vi "Update Slot Configuration.vi"(8 "error in (no error)":errorcluster, 9 "Card Position":T1[](array[typedef]) {"Slot #" max=15}, 10 "Card Name":string[](array[string]), 11 "Slot Configuration in":refnum<vi>) -> (0 "error out":errorcluster, 3 "Slot Configuration out":refnum<vi>)   [LabVIEW 2014, in "SLSC configuration System Explorer.lvlib"]
uses:
  SLSC configuration System Explorer.lvlib
  Type Defs/Card Position.ctl
  Example/SPI Utility/Slot #.ctl
  <vilib>/Utility/miscctls.llb/LVRowAndColumnTypeDef.ctl
  Shared/Constants.vi
  Shared/SLSC configuration Shared.lvlib
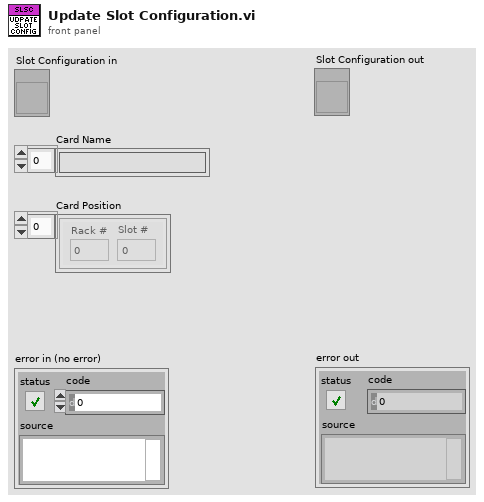
[diagram p1: front panel]
types:
  T1 = typedef "SLSC configuration Shared.lvlib/Card Position.ctl" = cluster{"Rack #":u8, "Slot #":T2}
  T2 = typedef "SLSC configuration Shared.lvlib/Slot #.ctl" = u8
  T3 = typedef "LVRowAndColumnTypeDef.ctl" = cluster{"Row":i32, "Column":i32}
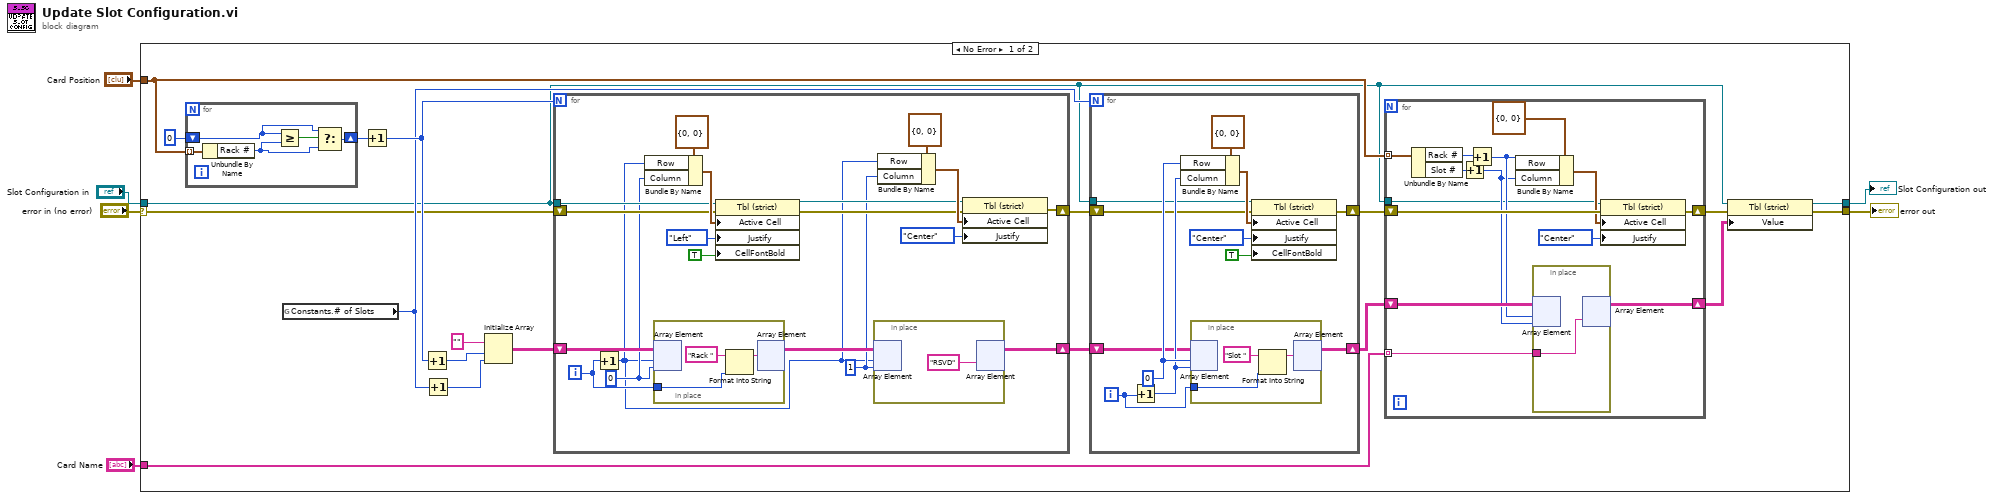
[diagram p0: block diagram]
diagram:
  n1 = case shown="No Error" "error in (no error)" {
    selector: "error in (no error)" -> [w12 w85]
    tunnel: "Card Position" -> [w23 _]
    tunnel: "Card Name" -> [w22 _]
    tunnel: [w10 w85] -> w1
    tunnel: "Slot Configuration in" -> [w7 w86]
    tunnel: [w8 w86] -> w2
    frame No Error {
      n2 = for {
        tunnel: w23 -> [w80] mode=indexing
        shift-right: [w81] -> w20
        shift-left: u8 0 ("Rack #") -> [w83]
        n3 = Unbundle By Name(w80) -> ("Rack #"=w82:u8)
        n4 = Greater Or Equal?(x=w83, y=w82) -> (x >= y?=w84:bool)
        n5 = Select(t=w83, s=w84, f=w82) -> (s? t:f=w81:u8)
      }
      n6 = global read "Constants.vi" "Constants.# of Slots"() -> (w13:u8)
      n7 = Increment(x=w20) -> (x+1=w19:u8)
      n8 = Increment(x=w19) -> (x+1=w24:u8)
      n9 = Increment(x=w13) -> (x+1=w14:u8)
      n10 = Initialize Array("", w24, w14) -> (w21:string[][])
      n11 = for {
        N: w19 -> [_]
        shift-right: [w43] -> w18
        shift-left: w21 -> [w60]
        shift-right: [w46] -> w17
        shift-left: w12 -> [w56]
        tunnel: w7 -> [w55]
        i -> [w45]
        w44 = 1
        w53 = 0
        n12 = Increment(x=w45) -> (x+1=w42:i32)
        n13 = Bundle By Name(cluster=T3 {"Row"=0, "Column"=0} ("Active Cell:Active Cell"), "Row"=w42, "Column"=w53) -> (w58:T3)
        n14 = in-place {
          in-place-border: w45 -> [w64]
          n15 = in-place-array #1(w60, w42, w53) -> ()  [unwired: 1 out]
          n16 = Format Into String(initial string="Rack ", w64) -> (resulting string=w62:string)  [unwired: 2 in, 1 out]
          n17 = in-place-array #1(w62) -> (w52:string[][])  [unwired: 2 out]
        }
        n18 = property class="Tbl (strict)"(reference=w55, error in=w56, "Active Cell"=w58, "Justify"=enum16{"Left", "Center", "Right"}."Left" ("Active Cell:Cell Justification"), "CellFontBold"=TRUE ("Active Cell:Cell Font:Bold")) -> (reference out=w47:refnum<vi>, error out=w48:errorcluster)
        n19 = in-place {
          n20 = in-place-array #2(w52, w42, w44) -> ()  [unwired: 1 out]
          n21 = in-place-array #2("RSVD" ("initial string")) -> (w43:string[][])  [unwired: 2 out]
        }
        n22 = Bundle By Name(cluster=T3 {"Row"=0, "Column"=0} ("Active Cell:Active Cell"), "Row"=w42, "Column"=w44) -> (w50:T3)
        n23 = property class="Tbl (strict)"(reference=w47, error in=w48, "Active Cell"=w50, "Justify"=enum16{"Left", "Center", "Right"}."Center" ("Active Cell:Cell Justification")) -> (error out=w46:errorcluster)  [unwired: 1 out]
      }
      n24 = for {
        N: w13 -> [_]
        shift-right: [w28] -> w16
        shift-left: w18 -> [w29]
        shift-right: [w27] -> w15
        shift-left: w17 -> [w31]
        tunnel: w7 -> [w30]
        i -> [w34]
        w33 = 0
        n25 = Increment(x=w34) -> (x+1=w32:i32)
        n26 = Bundle By Name(cluster=T3 {"Row"=0, "Column"=0} ("Active Cell:Active Cell"), "Row"=w33, "Column"=w32) -> (w37:T3)
        n27 = in-place {
          in-place-border: w34 -> [w41]
          n28 = in-place-array #3(w29, w33, w32) -> ()  [unwired: 1 out]
          n29 = Format Into String(initial string="Slot ", w41) -> (resulting string=w39:string)  [unwired: 2 in, 1 out]
          n30 = in-place-array #3(w39) -> (w28:string[][])  [unwired: 2 out]
        }
        n31 = property class="Tbl (strict)"(reference=w30, error in=w31, "Active Cell"=w37, "Justify"=enum16{"Left", "Center", "Right"}."Center" ("Active Cell:Cell Justification"), "CellFontBold"=TRUE ("Active Cell:Cell Font:Bold")) -> (error out=w27:errorcluster)  [unwired: 1 out]
      }
      n32 = for {
        tunnel: w23 -> [w77] mode=indexing
        shift-right: [w70] -> w9
        shift-left: w16 -> [w72]
        tunnel: w22 -> [w71] mode=indexing
        shift-right: [w73] -> w11
        shift-left: w15 -> [w78]
        tunnel: w7 -> [w65]
        n33 = Unbundle By Name(w77) -> ("Rack #"=w68:u8, "Slot #"=w69:T2)
        n34 = Increment(x=w69) -> (x+1=w66:T2)
        n35 = Increment(x=w68) -> (x+1=w67:u8)
        n36 = Bundle By Name(cluster=T3 {"Row"=0, "Column"=0} ("Active Cell:Active Cell"), "Row"=w67, "Column"=w66) -> (w75:T3)
        n37 = in-place {
          in-place-border: w71 -> [w79]
          n38 = in-place-array #4(w72, w67, w66) -> ()  [unwired: 1 out]
          n39 = in-place-array #4(w79) -> (w70:string[][])  [unwired: 2 out]
        }
        n40 = property class="Tbl (strict)"(reference=w65, error in=w78, "Active Cell"=w75, "Justify"=enum16{"Left", "Center", "Right"}."Center" ("Active Cell:Cell Justification")) -> (error out=w73:errorcluster)  [unwired: 1 out]
      }
      n41 = property class="Tbl (strict)"(reference=w7, error in=w11, "Value"=w9) -> (reference out=w8:refnum<vi>, error out=w10:errorcluster)
    }
    frame Error {
    }
  }
  "error out" <- w1
  "Slot Configuration out" <- w2
